vi "Mover4_Hand_Control_Stream_Connection_Full_System.vi"() -> ()   [LabVIEW 2015]
uses:
  <vilib>/Platform/TimedLoop/XDataNode/timing_clust.ctl
  <vilib>/Platform/TimedLoop/XDataNode/nitl_modes.ctl
  <vilib>/Platform/TimedLoop/XDataNode/wakeup.ctl
  <instrlib>/Dynamixel Motor/Public/Motor Operation/Low Level/Baud Setting.ctl
  <vilib>/Utility/miscctls.llb/LVRGBAColorTypeDef.ctl
  <vilib>/MakerHub/KinectOne/Private/Initialize Image [Color].vi
  Microsoft.Kinect
  C:/Program Files (x86)/National Instruments/LabVIEW 2015/vi.lib/MakerHub/KinectOne/Private/Libs/BodyFrameDataInterface.dll
  Program Files (x86)/National Instruments/LabVIEW 2015/vi.lib/MakerHub/KinectOne/Private/Libs/BodyFrameDataInterface.dll
  <vilib>/platform/TimedLoop/XDataNode/XDataNode.xnode
  <vilib>/robotics/Kinematics/Plotting/NI_Robotics_3DKinematics.lvlib
  <vilib>/MakerHub/KinectOne/KinectOne.lvlib
  <vilib>/Platform/TimedLoop/XDataNode/XDNodeRunTimeDep.lvlib
  <instrlib>/Dynamixel Motor/Dynamixel Motor.lvlib
  <vilib>/MakerHub/Leap/LMH-Leap.lvlib
panel:
  out "Simulation":refnum<vi>(3d-picture)
  out "Hand motors info":T1(array[cluster])
  out "Mover4 positions (degree)":T2(array[cluster]) {"Error Code (bits)" format="%b"}
  out "Camera output":T3(plugin-control)
  out "Stop?":bool
  in  "VISA resource name":refnum<visa-resource-name>="COM9"
  in  "Leap Calibrate?":bool
  out "Position Left Wrist (XYZ) detected by Kinect":dbl[](array[numeric])
  in  "Reset Mover4 To Zero?":bool
  out "Position not reachable?":bool=TRUE
  in  "Target IP Address":string="172.22.11.2"
  in  "Stop":bool
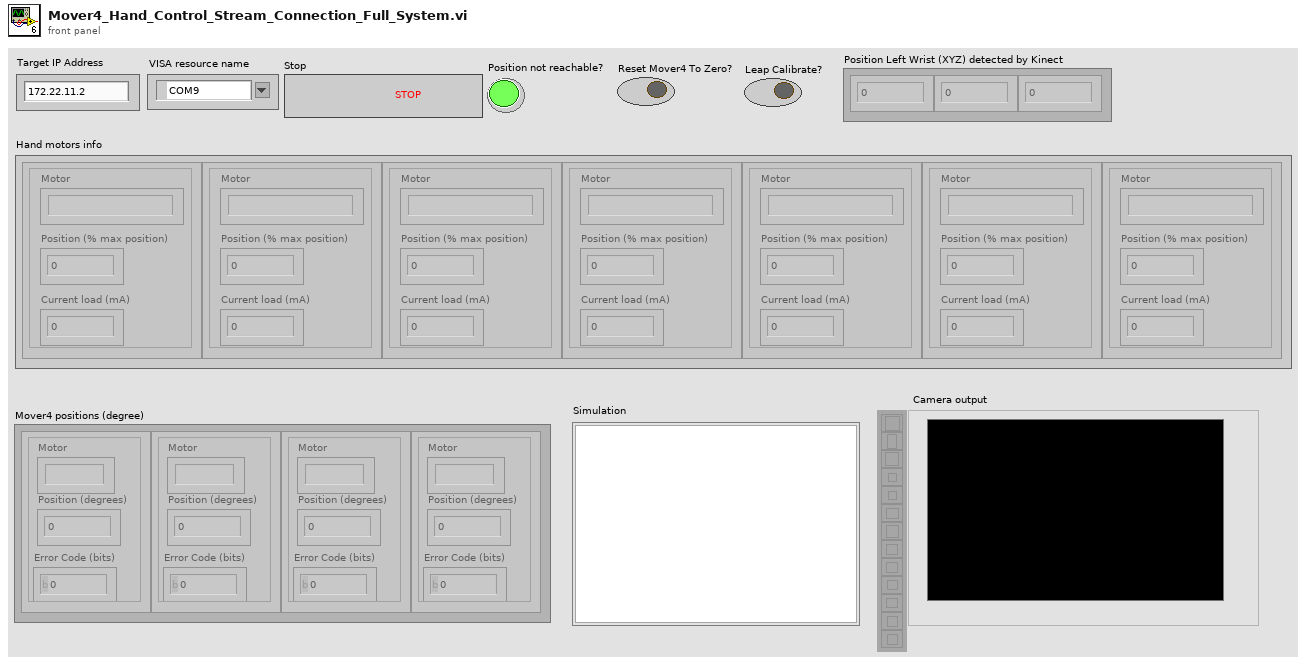
[diagram p1: front panel]
types:
  T1 = cluster{"Motor ":string, "Position (% max position)":dbl, "Current load (mA)":dbl}[]
  T2 = cluster{"Position (degrees)":i32, "Error Code (bits)":u8, "Motor":string}[]
  T3 = typedef "IMAQ Image.ctl" = refnum<image>
  T4 = typedef "LVRGBAColorTypeDef.ctl" = cluster{"Red":sgl, "Green":sgl, "Blue":sgl, "Alpha":sgl}
  T5 = typedef "Dynamixel Motor.lvlib/Baud Setting.ctl" = u8
  T6 = cluster{"Desired Position":u16, "Enable?":bool, "Reset?":bool}[]
  T7 = cluster{"ID":u8, "Position":u16, "Error Code":u8}[]
  T8 = cluster{"Read Access":enum8{"Allowed", "Required", "None"}, "Write Access":enum8{"Allowed", "Required", "None"}}
  T9 = typedef "LMH-Leap.lvlib/Leap Handle.ctl" = cluster{"LeapCSharp":refnum<k24>}
  T10 = cluster{"Motor ":string, "Position (% Max position)":dbl, "Current load (mA)":dbl}[]
  T11 = typedef "KinectOne.lvlib/KinectSensor References.ctl" = cluster{"KinectSensor":refnum<k24>, "MultiSourceFrameReader":refnum<k24>, "BodyFrameDataInterface":refnum<k24>}
  T12 = typedef "XDNodeRunTimeDep.lvlib/timing_clust.ctl" = cluster{"Expected End [f-1]":u64, "Actual End [f-1]":u64, "Finished Late? [f-1]":bool, "Expected End [i-1]":u64, "Actual End [i-1]":u64, "Finished Late? [i-1]":bool, "Expected Start [i]":u64, "Actual Start [i]":u64, "Expected Start [f]":u64, "Actual Start [f]":u64, "Source Name":string, "Structure Name":string, "Period":i64, "Deadline":i64, "Offset":i64, "Start":i64, "Priority":i32, "Timeout":i32, "Mode":T13, "Wakeup Reason":T14, "Error":errorcluster, "Source Type":string, "Secondary Source Type":string, "Global End Time":u64, "Global Start Time":u64, "Frame Duration":u64, "Iteration Duration":u64, "Assigned CPU":i32, "I/O Scan Engine Mode":u32}
  T13 = typedef "XDNodeRunTimeDep.lvlib/nitl_modes.ctl" = enum32{"No Change", "Process missed periods, maintain original phase", "Discard missed periods, maintain original phase", "Process missed periods, ignore original phase", "Discard missed periods, ignore original phase"}
  T14 = typedef "XDNodeRunTimeDep.lvlib/wakeup.ctl" = enum32{"Normal", "Aborted", "Asynchronous wakeup", "Timing source error", "Timed loop error", "Timeout"}
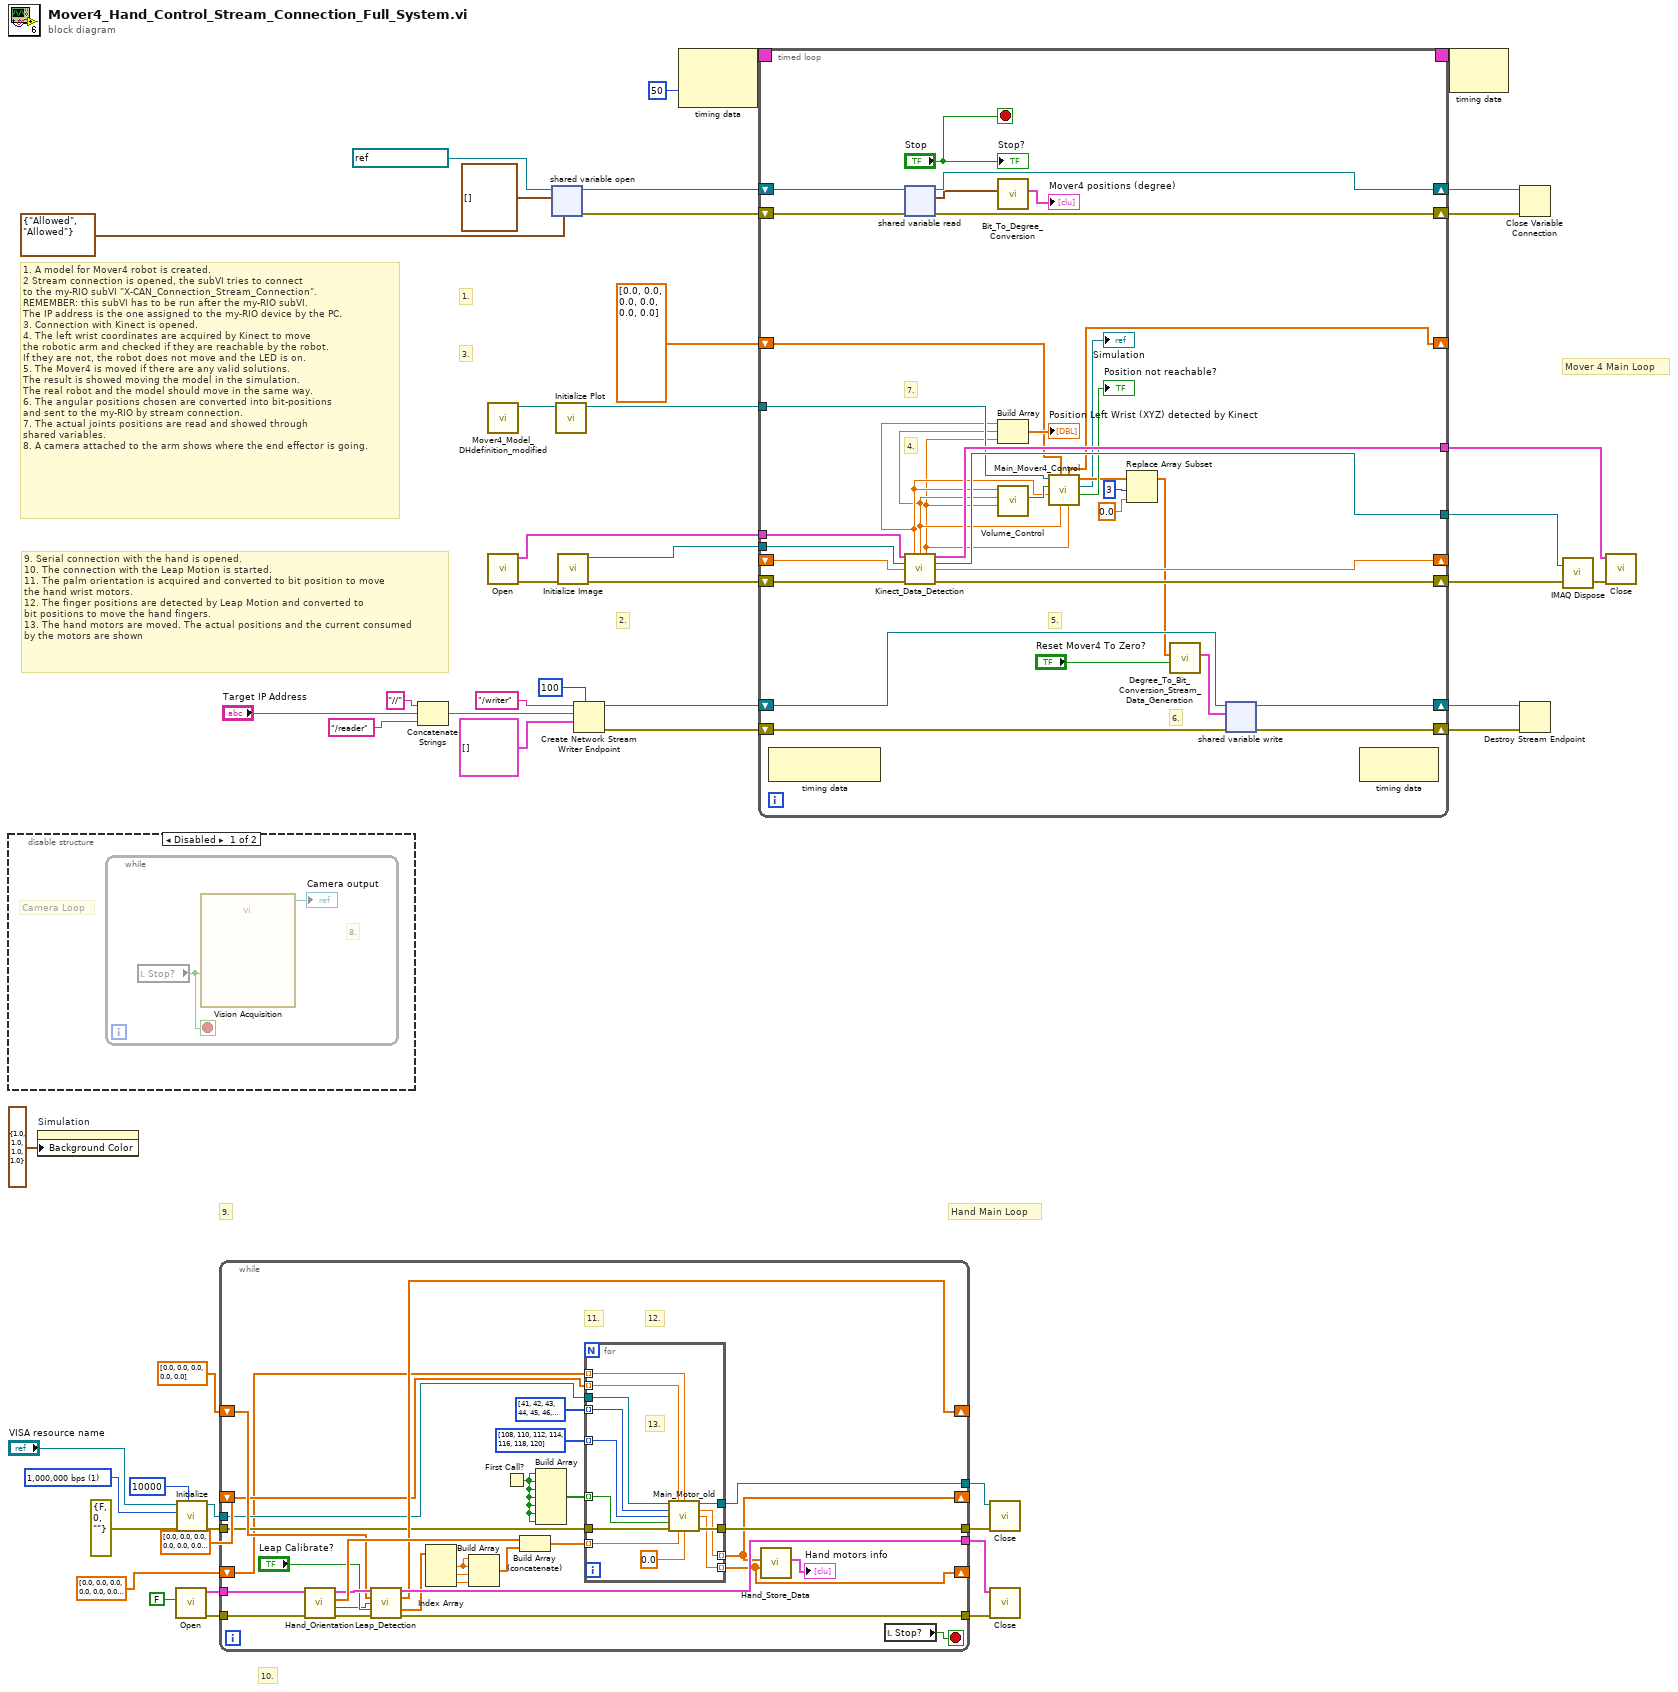
[diagram p0: block diagram]
diagram:
  w17 = T5 1 items=["1,000,000 bps"=1, "500,000 bps"=3, "400,000 bps"=4, "250,000 bps"=7, "200,000 bps"=9, "115200 bps"=16, "57600 bps"=34, "19200 bps"=103, "9600 bps"=207] ("Baud rate (57600 bps)")
  # "10."
  # "9."
  # "3."
  # "2."
  # "1."
  # "9. Serial connection with the hand is opened.\n10. The connection with the Leap Motion is started.\n11. The palm orientation is acquired and converted to bit position to move \nthe hand wrist motors.\n12. The finger positions are detected by Leap Motion and converted to\nbit positions to move the hand fingers.\n13. The hand motors are moved. The actual positions and the current consumed\nby the motors are shown"
  # "1. A model for Mover4 robot is created.\n2 Stream connection is opened, the subVI tries to connect\nto the my-RIO subVI \"X-CAN_Connection_Stream_Connection\".\nREMEMBER: this subVI has to be run after the my-RIO subVI. \nThe IP address is the one assigned to the my-RIO device by the PC.\n3. Connection with Kinect is opened.\n4. The left wrist coordinates are acquired by Kinect to move \nthe robotic arm and checked if they are reachable by the robot.\nIf they are not, the robot does not move and the LED is on.\n5. The Mover4 is moved if there are any valid solutions.\nThe result is showed moving the model in the simulation. \nThe real robot and the model should move in the same way.\n6. The angular positions chosen are converted into bit-positions\nand sent to the my-RIO by stream connection.\n7. The actual joints positions are read and showed through\nshared variables.\n8. A camera attached to the arm shows where the end effector is going."
  # "Hand Main Loop"
  # "Mover 4 Main Loop"
  n1 = disable-structure shown="Disabled" {
    frame Disabled {
      # "Camera Loop"
      n2 = while {
        stop <- w50 stop-if-true
        # "8."
        n3 = local read "Stop?"() -> (w50:bool)
        n4 = call "Vision Acquisition"("Stop (F)"=w50) -> ("Image Out"=→"Camera output":T3)  [unwired: 24 in, 2 out]
      }
    }
    frame Enabled {
    }
  }
  n5 = property on="Simulation" class="SceneGraphDisp (strict)"("Background Color"=T4 {"Red"=1.0, "Green"=1.0, "Blue"=1.0, "Alpha"=1.0}) -> ()  [unwired: 2 in, 2 out]
  n6 = call <vilib>:"Open.vi"("Enable Gestures? (T)"=FALSE) -> ("Error Out"=w9:errorcluster, "Leap Handle"=w10:T9)  [unwired: 9 in]
  n7 = call <instrlib>:"Initialize.vi"("Timeout (30 msec)"=u32 10000, "error in (no error)"=errorcluster {"status"=FALSE, "code"=0, "source"=""}, "Baud rate (57600 bps)"=w17, "VISA resource name"="VISA resource name") -> ("error out"=w12:errorcluster, "VISA resource name out"=w13:refnum<visa-resource-name>)  [unwired: 6 in]
  n8 = while {
    tunnel: w13 -> [w59]
    tunnel: w12 -> [w58]
    tunnel: w10 -> [w78]
    tunnel: w9 -> [w77]
    tunnel: [w72] -> w8
    shift-right: [w70] -> _
    shift-left: sgl[] [0.0, 0.0, 0.0, 0.0, 0.0] ("Max Distance out") -> [w68]
    tunnel: [w71] -> w6
    tunnel: [w57] -> w4
    tunnel: [w56] -> w3
    shift-right: [w53] -> _
    shift-left: dbl[] [0.0, 0.0, 0.0, 0.0, 0.0, 0.0, 0.0] -> [w55]
    shift-right: [w52] -> _
    shift-left: dbl[] [0.0, 0.0, 0.0, 0.0, 0.0, 0.0, 0.0] -> [w54]
    stop <- w75 stop-if-true
    # "12."
    # "11."
    n9 = call "Hand_Orientation.vi"("Error In"=w77, "Leap Handle in"=w78) -> ("Error Out"=w73:errorcluster, "Hand not tracked?"=w66:bool, "Palm Orientation"=w76:dbl[], "Leap Handle"=w74:T9)  [unwired: 6 in]
    n10 = call "Leap_Detection.vi"("Leap Handle in"=w74, "Max distance in"=w68, "Not Tracked?"=w66, "Calibrate?"="Leap Calibrate?", "error in (no error)"=w73) -> ("Leap Handle out"=w71:T9, "Max Distance out"=w70:dbl[], "Finger Positions"=w69:dbl[], "error out"=w72:errorcluster)  [unwired: 7 in]
    n11 = Index Array(array=w69) -> (element #1=w82:dbl, element #2=w81:dbl, element #3=w80:dbl)  [unwired: 3 in]
    n12 = Build Array(w82, w82, w81, w80) -> (w79:dbl[])
    n13 = First Call?() -> (First Call?: T/F=w64:bool)
    n14 = Build Array (concatenate)(w76, w79) -> (w60:dbl[])
    n15 = Build Array(w64, w64, w64, w64, w64, w64, w64) -> (w63:bool[])
    n16 = for {
      tunnel: [w95] -> w56
      tunnel: [w94] -> w57
      tunnel: [w93] -> w53 mode=indexing
      tunnel: [w92] -> w52 mode=indexing
      tunnel: w63 -> [w91] mode=indexing
      tunnel: u8[] [41, 42, 43, 44, 45, 46, 47] ("Motor ID") -> [w89] mode=indexing
      tunnel: u8[] [108, 110, 112, 114, 116, 118, 120] ("Address # DEC") -> [w88] mode=indexing
      tunnel: w60 -> [w87] mode=indexing
      tunnel: w59 -> [w86]
      tunnel: w58 -> [w85]
      tunnel: w55 -> [w84] mode=indexing
      tunnel: w54 -> [w83] mode=indexing
      # "13."
      n17 = call "Main_Motor_old.vi"("VISA resource name"=w86, "Old Position Motor"=w84, "Old Current load"=w83, "Motor ID"=w89, "Address"=w88, "Torque enable?"=w91, "error in (no error)"=w85, "Goal Position"=w87, "Goal Speed (RPM)"=0.0) -> ("VISA resource name out"=w94:refnum<visa-resource-name>, "New Position Motor"=w93:dbl, "New Current load (mA)"=w92:dbl, "error out"=w95:errorcluster)  [unwired: 3 in]
    }
    n18 = call "Hand_Store_Data.vi"("Current load (mA)"=w52, "Position (bits)"=w53) -> ("Motors info"=→"Hand motors info":T10)  [unwired: 9 in]
    n19 = local read "Stop?"() -> (w75:bool)
  }
  n20 = Concatenate Strings("//", "Target IP Address", "/reader") -> (w42:string)
  n21 = call "Mover4_Model_DHdefinition_modified.vi"() -> ("serial arm out"=w29:refnum<class "NI_Robotics_6R Type 1 Serial Arm Class.lvclass">)  [unwired: 10 in, 1 out]
  n22 = call <vilib>:"Open.vi"() -> ("Error Out"=w28:errorcluster, "KinectSensor References out"=w27:T11)  [unwired: 10 in]
  n23 = shared-variable-open(refnum<k21> "ni.var.psp://stratom-myrio/Shared_Variables/New position" ("shared variable refnum in"), T7 [] ("New position 2"), T8 {"Read Access"=enum."Allowed", "Write Access"=enum."Allowed"} ("access")) -> (w49:refnum<k21>, w48:errorcluster)  [unwired: 1 in]
  n24 = call <vilib>:"Initialize Plot.vi"("serial arm in"=w29) -> ("serial arm out"=w30:refnum<class "NI_Robotics_6R Type 1 Serial Arm Class.lvclass">)  [unwired: 9 in, 1 out]
  n25 = call-poly <vilib>:"Initialize Image.vi"("Error In"=w28) -> ("Error Out"=w26:errorcluster, "Color Image"=w25:T3)  [unwired: 9 in]
  n26 = Create Network Stream Writer Endpoint(7:100 ("writer buffer size"), 9:T6 [] ("Commands 2"), 10:w42, 11:"/writer" ("reader name")) -> (0:w35:errorcluster, 3:w36:refnum<k21>)  [unwired: 3 in]
  n27 = node-c288(i64 50 ("Period")) -> (w20:T12)  [unwired: 1 in]
  n28 = timed-loop {
    shift-right: [w128] -> w45
    shift-left: w49 -> [w130]
    shift-right: [w127] -> w44
    shift-left: w48 -> [w129]
    shift-right: [w124] -> w34
    shift-left: w36 -> [w126]
    shift-right: [w123] -> w33
    shift-left: w35 -> [w125]
    shift-right: [w103] -> _
    shift-left: dbl[] [0.0, 0.0, 0.0, 0.0, 0.0, 0.0] ("current joint positions") -> [w105]
    tunnel: w30 -> [w110]
    tunnel: w27 -> [w120]
    tunnel: w25 -> [w119]
    shift-right: [w115] -> w23
    shift-left: w26 -> [w118]
    tunnel: [w117] -> w22
    tunnel: [w116] -> w21
    shift-right: [w112] -> _
    shift-left: _ -> [w113]
    timing: w20 -> [_]
    timing-out: [_] -> w19
    stop <- "Stop" stop-if-true
    # "7."
    # "6."
    # "5."
    # "4."
    n29 = node-c288() -> ()  [unwired: 1 in, 1 out]
    n30 = shared-variable-read(w130, w129) -> (w128:refnum<k21>, w127:errorcluster, w98:T7)  [unwired: 1 out]
    n31 = call "Kinect_Data_Detection.vi"("KinectSensor References in"=w120, "Image"=w119, "Distance from Kinect (m)"=w113, "error in (no error)"=w118) -> ("X (m)"=w108:dbl, "Y (m)"=w107:dbl, "Z (m)"=w106:dbl, "KinectSensor References"=w116:T11, "Image Out"=w117:T3, "Distance from Kinect (calibrated, m)"=w112:dbl, "Error Out"=w115:errorcluster)  [unwired: 5 in]
    n32 = call "Bit_To_Degree_Conversion.vi"("Actual joints positions"=w98) -> ("Motor positions (degree)"=→"Mover4 positions (degree)":T2)  [unwired: 10 in]
    n33 = Build Array(w108, w107, w106) -> (→"Position Left Wrist (XYZ) detected by Kinect":dbl[])
    n34 = call "Volume_Control.vi"("z (m)"=w106, "y (m)"=w107, "x (m)"=w108) -> ("Range acceptable?"=w109:bool)  [unwired: 8 in]
    n35 = call "Main_Mover4_Control.vi"("Z (m)"=w106, "Y (m)"=w107, "current joint positions in"=w105, "X (m)"=w108, "Range acceptable?"=w109, "NI_Robotics_6R Type 1 Serial Arm Class in"=w110) -> ("Position not reachable?"=→"Position not reachable?":bool, "Simulation"=→"Simulation":refnum<vi>, "current joint positions degree"=w102:dbl[], "current joint positions out"=w103:dbl[])  [unwired: 2 in]
    n36 = Replace Array Subset(array=w102, new element=0.0 ("new element/subarray"), index=3) -> (w99:dbl[])
    n37 = call "Degree_To_Bit_Conversion_Stream_Data_Generation.vi"("Reset To Zero?"="Reset Mover4 To Zero?", "Degree"=w99) -> ("Commands"=w122:T6)  [unwired: 9 in]
    n38 = shared-variable-write(w126, w125, w122) -> (w124:refnum<k21>, w123:errorcluster)  [unwired: 1 in, 1 out]
    n39 = node-c288() -> ()  [unwired: 1 in, 1 out]
    "Stop?" <- "Stop"
  }
  n40 = call <vilib>:"Close.vi"("error in (no error)"=w3, "VISA resource name"=w4) -> ()  [unwired: 9 in, 1 out]
  n41 = call <vilib>:"Close.vi"("Error In"=w8, "Leap Handle"=w6) -> ()  [unwired: 9 in, 1 out]
  n42 = node-c288(w19) -> ()  [unwired: 1 out]
  n43 = Close Variable Connection(8:w44, 11:w45) -> ()  [unwired: 1 out]
  n44 = Destroy Stream Endpoint(8:w33, 11:w34) -> ()  [unwired: 1 out]
  n45 = call "IMAQ Dispose"("Image"=w22, "error in (no error)"=w23) -> ("error out"=w24:errorcluster)  [unwired: 4 in]
  n46 = call <vilib>:"Close.vi"("Error In"=w24, "KinectSensor References"=w21) -> ()  [unwired: 9 in, 1 out]
